vi "get_component_type_name.vi"(8 "error in (no error)":errorcluster, 11 "GenericSweep in":refnum<class "GenericSweep.lvclass">) -> (0 "error out":errorcluster, 2 "component type":string="Sweep", 3 "GenericSweep out":refnum<class "GenericSweep.lvclass">)   [LabVIEW 2010, in "GenericSweep.lvclass"]
uses:
  GenericSweep.lvclass
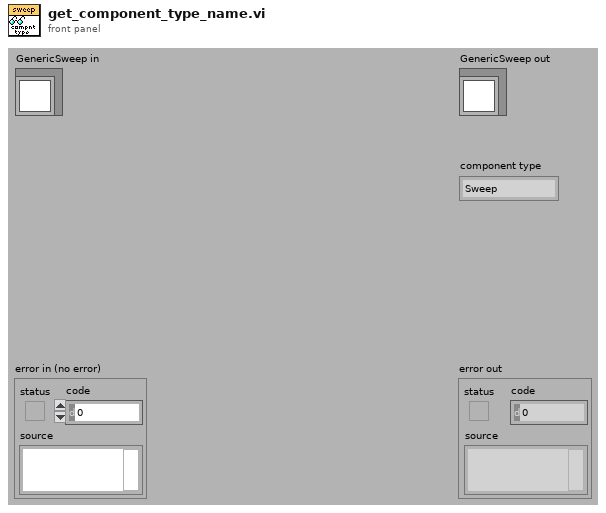
[diagram p1: front panel]
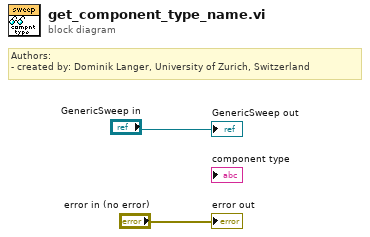
[diagram p0: block diagram]
diagram:
  # "Authors: \n- created by: Dominik Langer, University of Zurich, Switzerland"
  "error out" <- "error in (no error)"
  "GenericSweep out" <- "GenericSweep in"
